vi "Unix_time_to_Tclock.vi"(9 "Unix epoch zerotime (nanoseconds)":u64, 11 "Unix Timestamps (nanoseconds)":u64[](array[numeric])) -> (3 "Timestamps (seconds from T0)":dbl[](array[numeric]) format="%#.42g")   [LabVIEW 2021, in "Ring Buffer Strict Accessor.lvlib" / "Unix time epoch.lvlib"]
uses:
  Unix time epoch.lvlib
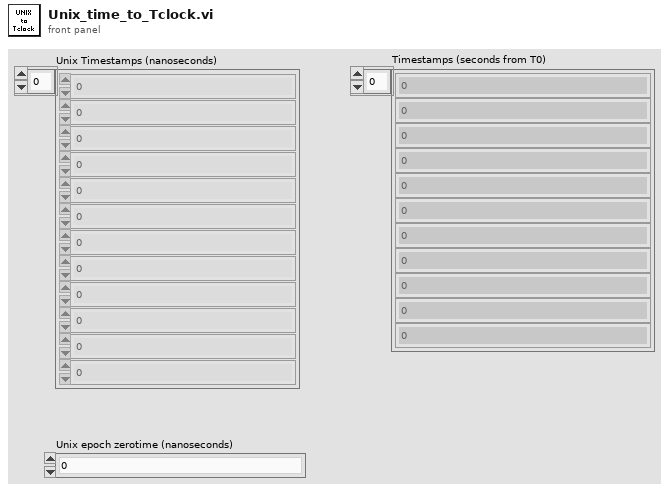
[diagram p1: front panel]
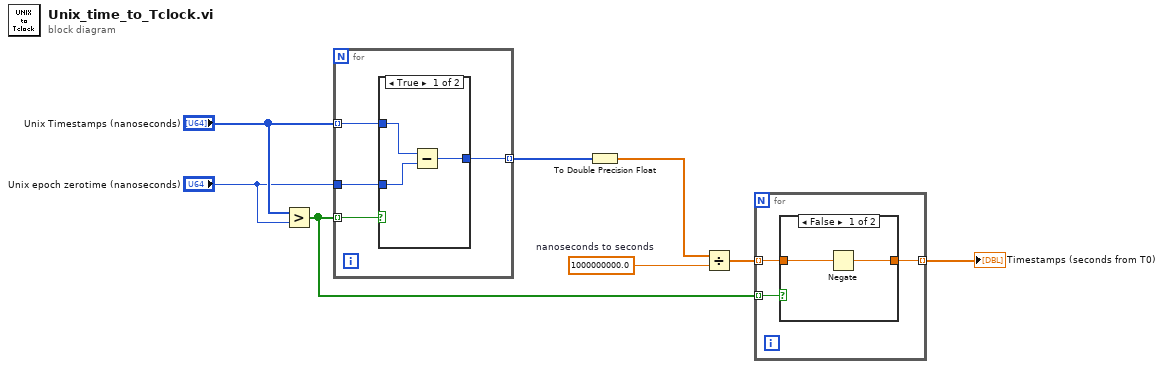
[diagram p0: block diagram]
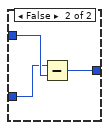
[diagram p3: hidden frame]
diagram:
  w5 = 1000000000.0  # nanoseconds to seconds
  n1 = Greater?(x="Unix Timestamps (nanoseconds)", y="Unix epoch zerotime (nanoseconds)") -> (0:w4:bool[])
  n2 = for {
    tunnel: [w12] -> w6 mode=indexing
    tunnel: "Unix Timestamps (nanoseconds)" -> [w11] mode=indexing
    tunnel: "Unix epoch zerotime (nanoseconds)" -> [w10]
    tunnel: w4 -> [w9] mode=indexing
    n3 = case shown="True" w9 {
      tunnel: [w15 w18] -> w12
      tunnel: w11 -> [w14 w17]
      tunnel: w10 -> [w13 w16]
      frame True {
        n4 = Subtract(x=w14, y=w13) -> (x-y=w15:u64)
      }
      frame False {
        n5 = Subtract(x=w16, y=w17) -> (x-y=w18:u64)
      }
    }
  }
  n6 = To Double Precision Float(number=w6) -> (double precision float=w1:dbl[])
  n7 = Divide(x=w1, y=w5) -> (x/y=w3:dbl[])
  n8 = for {
    tunnel: w4 -> [w21] mode=indexing
    tunnel: w3 -> [w20] mode=indexing
    tunnel: [w19] -> w2 mode=indexing
    n9 = case shown="False" w21 {
      tunnel: w20 -> [w23 w24]
      tunnel: [w22 w24] -> w19
      frame False {
        n10 = Negate(x=w23) -> (-x=w22:dbl)
      }
      frame True {
      }
    }
  }
  "Timestamps (seconds from T0)" <- w2
